vi "Create-message.vi"(8 "error in (no error)":errorcluster, 10 "Message type":T1) -> (0 "error out":errorcluster, 2 "Message out":refnum<class "Message.lvclass">)   [LabVIEW 2013, in "Client.lvlib" / "Client.lvclass"]
doc: "Creates a message object of the selected type and wraps this in the base 'Message' object.\nThis function also sets the 'Type' property of the message object to the selected type.\n\nA 'Not implemented' error is returned if the selected type has no associated message object."
uses:
  Client.lvclass
  Messages/Sources/Message.lvclass
  Supported-messages.ctl
  Messages/Sources/Heartbeat/Heartbeat.lvclass
  Custom-errors.ctl
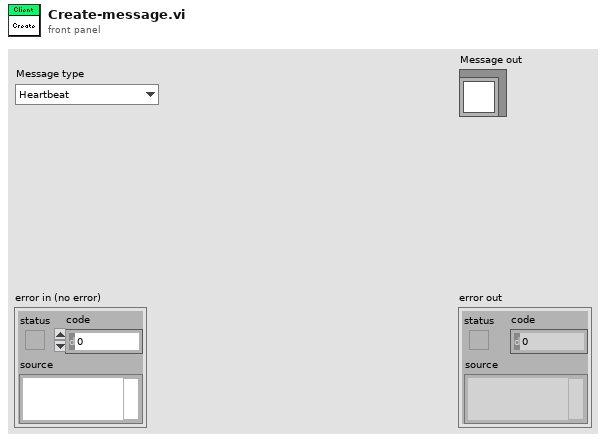
[diagram p1: front panel]
types:
  T1 = typedef "Client.lvlib/Client.lvclass/Supported-messages.ctl" = enum16{"Heartbeat", "Error", "Start client", "Client stopped", "Action", "Query status", "Send status", "Get clients"}
  T2 = typedef "Client.lvlib/Client.lvclass/Custom-errors.ctl" = enum16{"No error", "Command not recognized", "Invalid input", "Timeout", "Not implemented", "Unsupported message", "Unsupported client", "Unsupported action"}
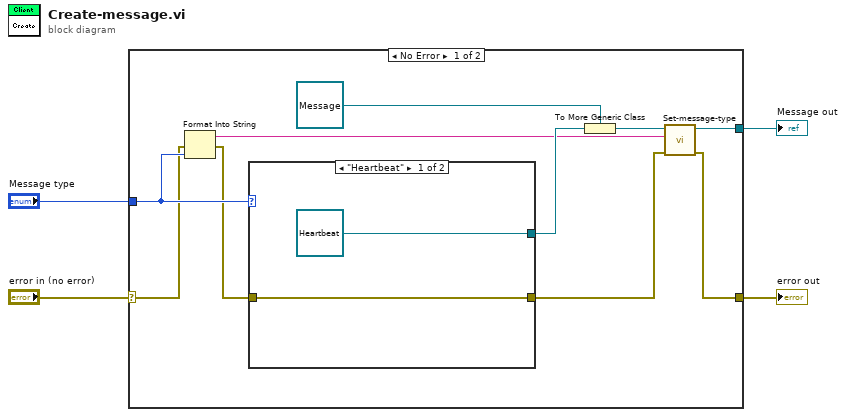
[diagram p0: block diagram]
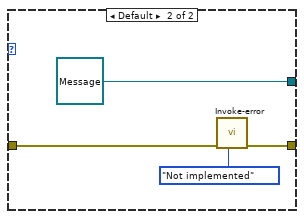
[diagram p2: hidden frame]
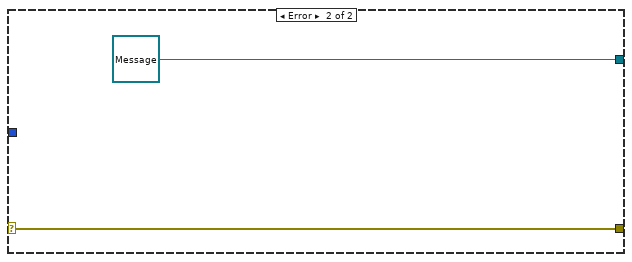
[diagram p3: hidden frame]
diagram:
  n1 = case shown="No Error" "error in (no error)" {
    selector: "error in (no error)" -> [w11 w22]
    tunnel: [w6 w22] -> w3
    tunnel: [w8 refnum<class "Message.lvclass"> refnum ("Module-communication.lvlib:Message.lvclass")] -> w2
    tunnel: "Message type" -> [w12 _]
    frame No Error {
      n2 = Format Into String(error in=w11, w12) -> (resulting string=w7:string, error out=w10:errorcluster)  [unwired: 2 in]
      n3 = case shown="\"Heartbeat\"" w12 {
        tunnel: w10 -> [w16 w19]
        tunnel: [w16 w18] -> w5
        tunnel: [refnum<class "Heartbeat.lvclass"> refnum ("Module-communication.lvlib:Heartbeat.lvclass") refnum<class "Message.lvclass"> refnum ("Module-communication.lvlib:Message.lvclass")] -> w14
        frame "Heartbeat" {
        }
        frame Default {
          n4 = call "Invoke-error.vi"("Error"=Custom-errors."Not implemented", "error in (no error)"=w19) -> ("error out"=w18:errorcluster)  [unwired: 9 in]
        }
      }
      n5 = To More Generic Class(target class=refnum<class "Message.lvclass"> refnum ("Module-communication.lvlib:Message.lvclass"), reference=w14) -> (generic class reference=w9:refnum<class "Message.lvclass">)
      n6 = call-dynamic "Set-message-type.vi"("error in (no error)"=w5, "Message type"=w7, "Message in"=w9) -> ("error out"=w6:errorcluster, "Message out"=w8:refnum<class "Message.lvclass">)  [unwired: 7 in]
    }
    frame Error {
    }
  }
  "error out" <- w3
  "Message out" <- w2
